vi "HolDrvCtrl_PackExecuteSP.vi"(8 "LinearVel":dbl=0.02, 9 "Heading_Deg":dbl=0.02, 10 "Y":dbl=0.02, 11 "X":dbl=0.02) -> (3 "HolExecuteSP":cluster{"DesiredPose":T1, "LinearVel":dbl} {"DesiredPose"."ROTATION"."SIN" format="%13.4f"; "DesiredPose"."ROTATION"."COS" format="%13.4f"; "DesiredPose"."ROTATION"."VALUE" format="%13.4f"; "DesiredPose"."TRANSLATION"."Y" format="%14.3f"; "DesiredPose"."TRANSLATION"."X" format="%14.3f"})   [LabVIEW 2019, in "Trajectory_Library.lvlib"]
doc: "Convience, single call, LabVIEW function. Packs individual values into a cluster to feed to the Holonomic controller execute function.\n\n \nInputs:\n - X -- X part of desired position\n - Y -- Y part f desired position\n - Heading_Deg -- Travel heading angle part of desired position (Degrees)\n - LinearVel -- Velocity in the direction of heading.\n\nOutputs:\n - HolExecuteSP -- Setpoint (desired position and velocity) to feed to Holonomic Execute function."
uses:
  Trajectory_Library.lvlib
  TRANSLATION2D.ctl
  ROTATION2D.ctl
  POSE2D.ctl
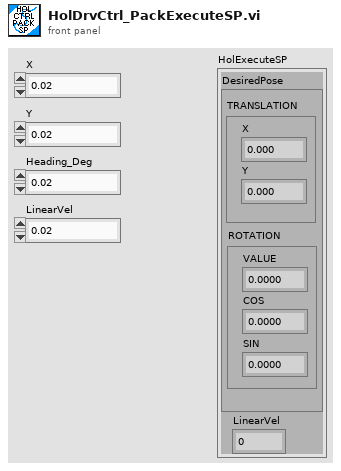
[diagram p1: front panel]
types:
  T1 = typedef "Trajectory_Library.lvlib/POSE2D.ctl" = cluster{"TRANSLATION":T2, "ROTATION":T3}
  T2 = typedef "Trajectory_Library.lvlib/TRANSLATION2D.ctl" = cluster{"X":dbl, "Y":dbl}
  T3 = typedef "Trajectory_Library.lvlib/ROTATION2D.ctl" = cluster{"VALUE":dbl, "COS":dbl, "SIN":dbl}
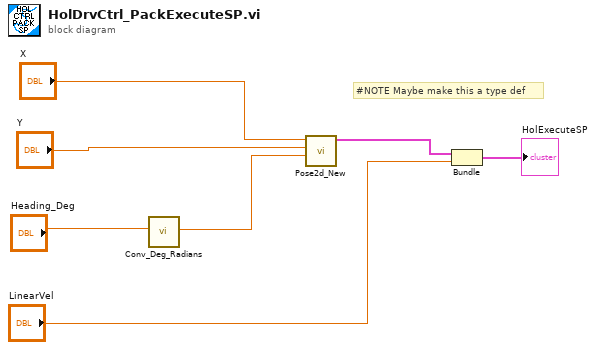
[diagram p0: block diagram]
diagram:
  # "#NOTE Maybe make this a type def"
  n1 = call "Conv_Deg_Radians.vi"("Degress"="Heading_Deg") -> ("Radians"=w4:dbl)  [unwired: 10 in]
  n2 = call "Pose2d_New.vi"("Heading"=w4, "Y"="Y", "X"="X") -> ("out POSe"=w3:T1)  [unwired: 8 in]
  n3 = Bundle("out POSe"=w3, "LinearVel"="LinearVel") -> (→"HolExecuteSP":cluster{"out POSe":T1, "LinearVel":dbl})  [unwired: 1 in]
